vi "St temp.vi"(11 "Station Name":string) -> ()   [LabVIEW 2019]
uses:
  Ctrl/Conveyor Action.ctl
  <vilib>/Utility/miscctls.llb/LVPointTypeDef.ctl
  LLB/Message/Ctrl/MsgDataInput.ctl
  LLB/Message/Ctrl/MsgPageSelect.ctl
  LLB/Message/Ctrl/LogType.ctl
  Ctrl/Auto Inspection Station Name2.ctl
  Ctrl/Auto Inspection Data Name.ctl
  ab69a899-d2ec-4c26-af5e-ed1cd18d461c.vi
  9b7d8055-4de2-48cf-bbcb-f861e34e7884.vi
  2931b48d-cced-43b2-9067-584d882f955d.vi
  Function/Axis/Axis_Class/SubVI/Axis Motion/Axis_Go Home.vi
  <vilib>/JDP Science/JSONtext/JSON text to Variant.vi
  <vilib>/JDP Science/JSONtext/Variant to JSON Text.vi
  LLB/Commonly VI.lvlib
  LLB/Message/MsgShowAndLog.lvlib
panel:
  in  "Btn_Home":bool
  in  "AI":T1
  in  "Tab Control":enum32{"Page 1", "Page 2"}(tab)
  in  "CurrentAction":string
  in  "Status":string
  in  "Errset":bool
  out "Message":string
  out "Ring":u16(ring)
  in  "Btn_AutoRun":bool
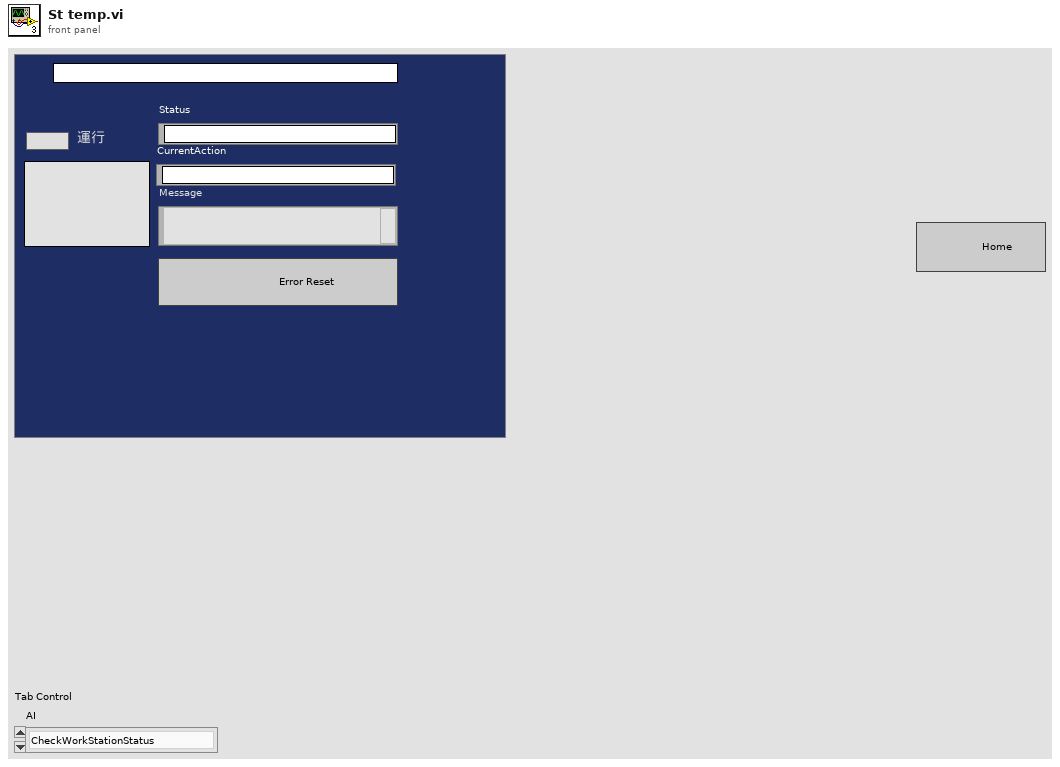
[diagram p1: front panel]
types:
  T1 = typedef "Conveyor Action.ctl" = enum16{"CheckWorkStationStatus", "Request Item In", "Check Product Ready In", "Wait Item In", "Check SlowSignal And Slow", "Check Arrive", "Rise Tray", "FixTray", "Imform Robot", "Wait Robot Imform", "DropTray Imform Out", "Wait Request ", "Flow Out"}
  T2 = enum8{"Enabled", "Disabled", "Disabled and Grayed Out"}
  T3 = typedef "LVPointTypeDef.ctl" = cluster{"Horizontal":i16, "Vertical":i16}
  T4 = typedef "MsgDataInput.ctl" = cluster{"MsgPageSelect":T5, "LogType":T6, "Msg":string, "Time":string}
  T5 = typedef "MsgShowAndLog.lvlib/MsgPageSelect.ctl" = enum16{"System", "Comm", "IO", "Action", "Alarm"}
  T6 = typedef "MsgShowAndLog.lvlib/LogType.ctl" = enum16{"Auto", "Manual", "Handshake", "Error"}
  T7 = typedef "Auto Inspection Station Name2.ctl" = enum16{"S1Barcode", "S2Measure", "S3Measure", "S4Measure", "S5Measure", "S11_LaserCheck", "S8_Vision AI"}
  T8 = typedef "Auto Inspection Data Name.ctl" = enum16{"LocalRun", "ItemSN(TimeCode)", "CurrentAction", "Error", "Data", "OKNG", "電壓值", "電壓值判斷", "電流值", "電流值判斷", "Laser1 Data", "Laser2 Data", "Laser OKNG", "StationNO"}
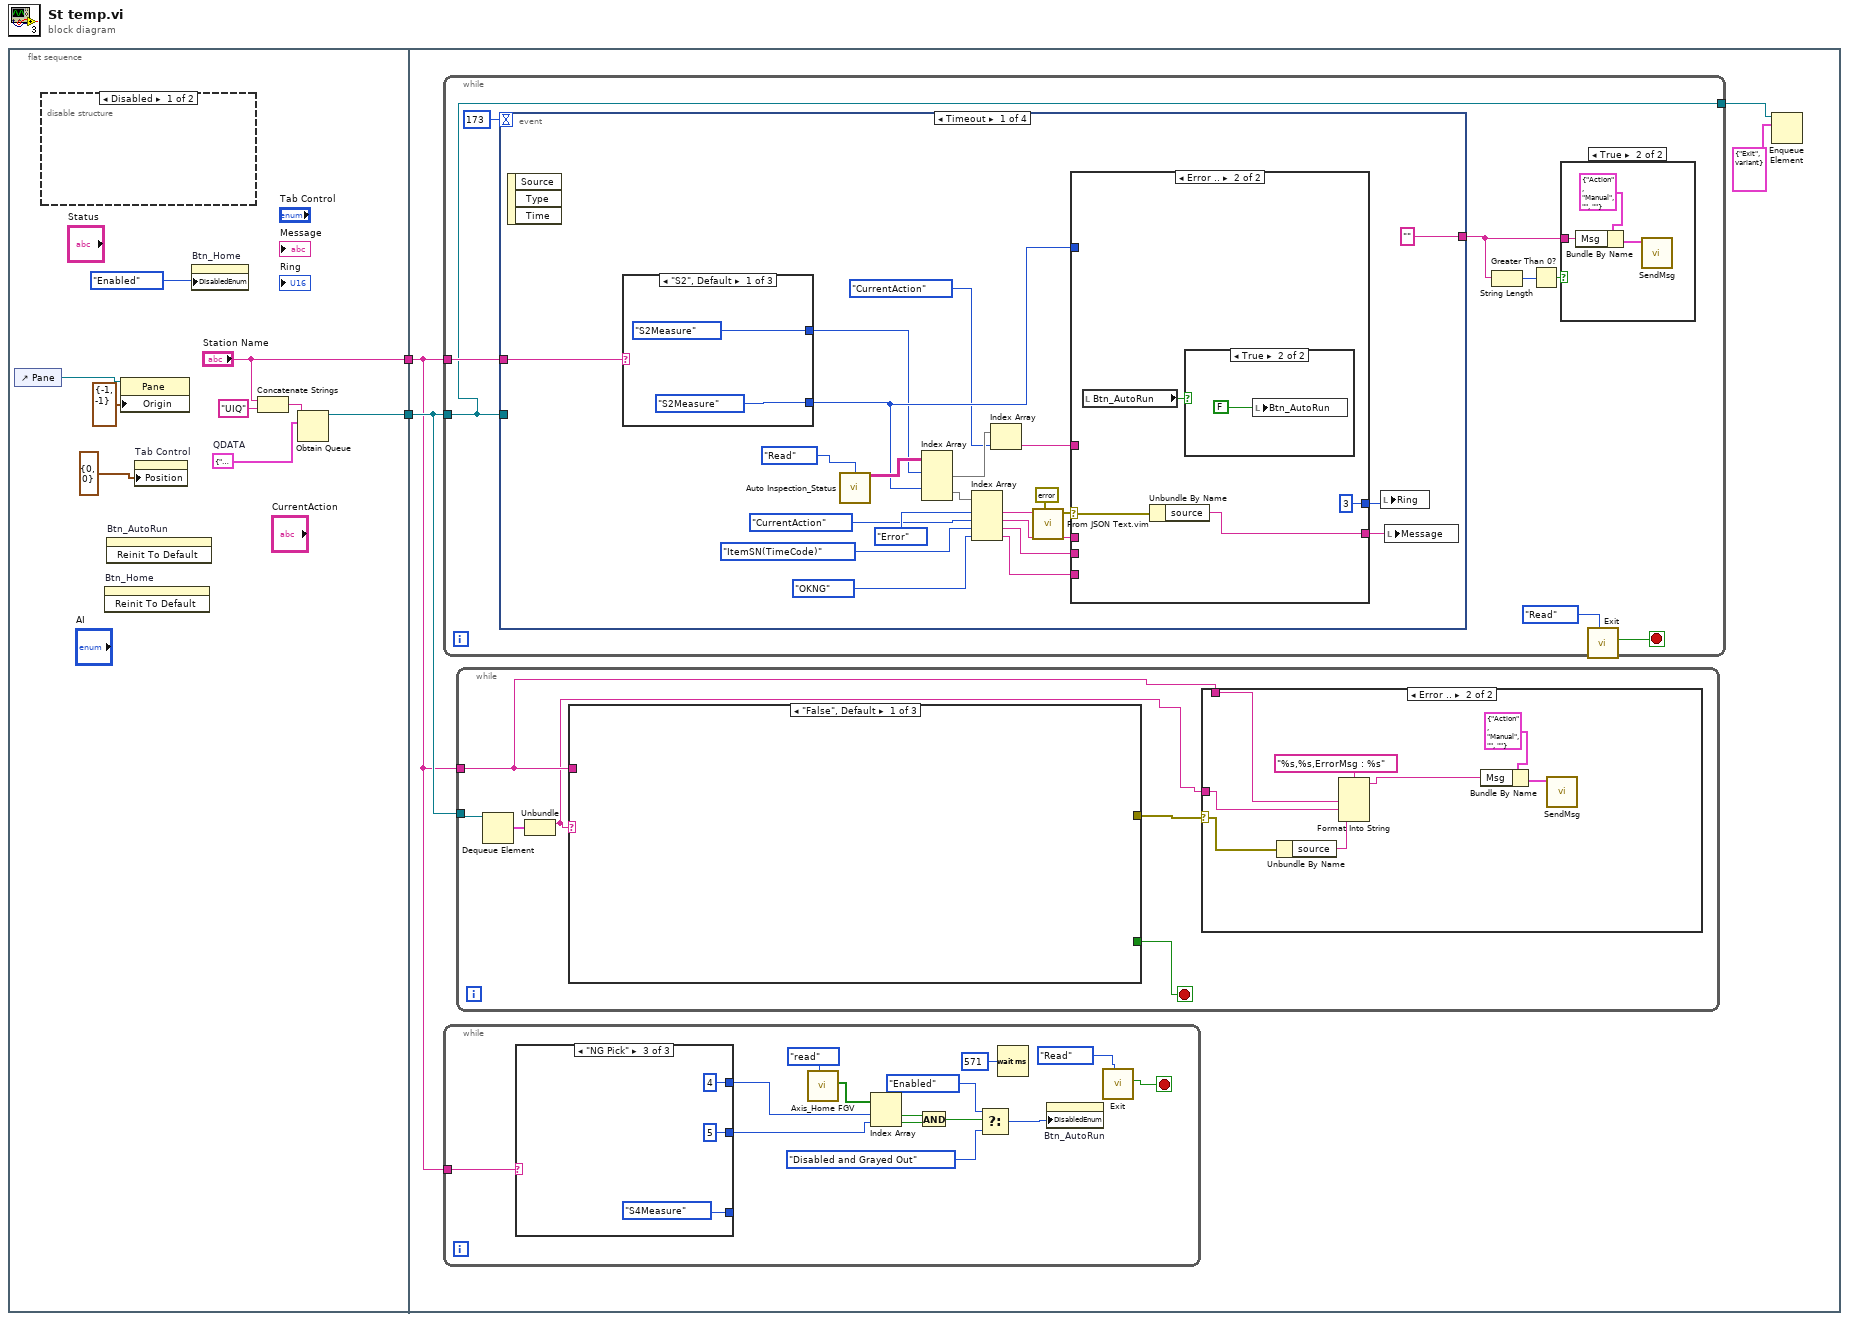
[diagram p0: block diagram]
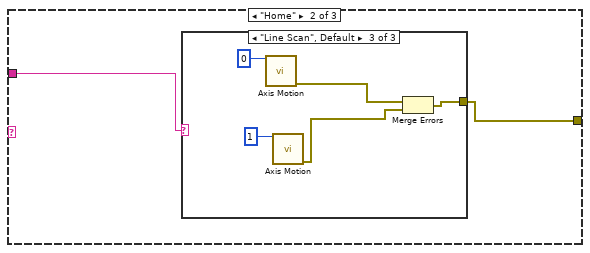
[diagram p4: hidden frame]
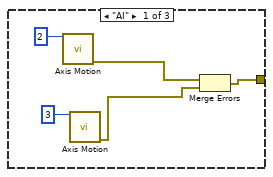
[diagram p5: hidden frame]
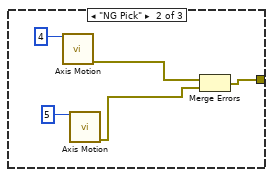
[diagram p6: hidden frame]
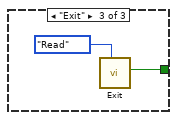
[diagram p7: hidden frame]
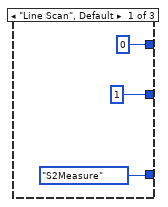
[diagram p8: hidden frame]
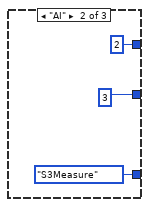
[diagram p9: hidden frame]
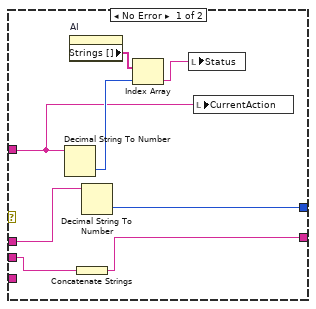
[diagram p11: hidden frame]
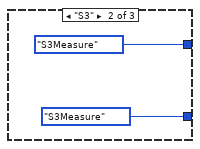
[diagram p13: hidden frame]
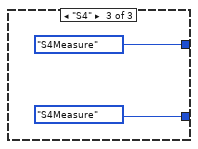
[diagram p14: hidden frame]
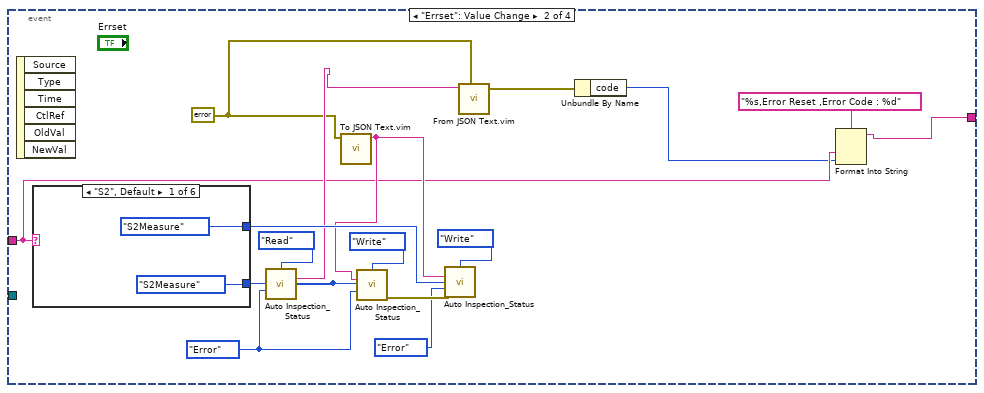
[diagram p15: hidden frame]
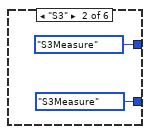
[diagram p16: hidden frame]
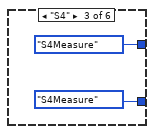
[diagram p17: hidden frame]
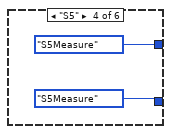
[diagram p18: hidden frame]
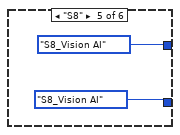
[diagram p19: hidden frame]
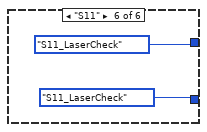
[diagram p20: hidden frame]
diagram:
  n1 = flat-sequence {
    tunnel: ["Station Name"] -> w2
    tunnel: [w3] -> w1
    tunnel: w2 -> [w12]
    tunnel: w1 -> [w15]
    frame #0 {
      w4 = cluster{"ACT":string, "DATA":variant} {"ACT"="", "DATA"=variant}  # QDATA
      n2 = control-ref of="Pane"() -> (w11:refnum<vi>)
      n3 = disable-structure shown="Disabled" {
        frame Disabled {
        }
        frame Enabled {
        }
      }
      n4 = invoke on="Btn_Home" class="Bool" method="Reinit To Default"() -> ()  [unwired: 3 in, 3 out]
      n5 = invoke on="Btn_AutoRun" class="Bool (strict)" method="Reinit To Default"() -> ()  [unwired: 3 in, 3 out]
      n6 = property class="Pane"(reference=w11, "Origin"=T3 {"Horizontal"=-1, "Vertical"=-1}) -> ()  [unwired: 1 in, 2 out]
      n7 = property on="Tab Control" class="TabCtl (strict)"("Position"=T3 {"Horizontal"=0, "Vertical"=0} ("Origin")) -> ()  [unwired: 2 in, 2 out]
      n8 = property on="Btn_Home" class="Bool"("DisabledEnum"=T2."Enabled" ("Disabled")) -> ()  [unwired: 2 in, 2 out]
      n9 = Concatenate Strings("Station Name", "UIQ" ("string")) -> (w5:string)
      n10 = Obtain Queue(name (unnamed)=w5, element data type=w4) -> (queue out=w3:refnum<queue>)  [unwired: 3 in, 2 out]
    }
    frame #1 {
      n11 = while {
        tunnel: w12 -> [w76]
        tunnel: w15 -> [w75]
        tunnel: [w75] -> w14
        stop <- w78 stop-if-true
        n12 = event shown="[0] Timeout" {
          selector: _ -> [_ _ _ _]
          dyn-events: _ -> [_ _ _ _]
          timeout: 173 -> [_ _ _ _]
          tunnel: w76 -> [w103 w126 w153 w186]
          tunnel: w75 -> [_ _ _ w185]
          tunnel: ["" w124 w155 w188] -> w74
          event Timeout {
            n13 = event-data() -> ()  [unwired: 1 in, 3 out]
            n14 = case shown="\"S2\", Default" w103 {
              tunnel: [Auto_Inspection_Station_Name2."S2Measure" ("Station") Auto_Inspection_Station_Name2."S3Measure" ("Station") Auto_Inspection_Station_Name2."S4Measure" ("Station")] -> w89
              tunnel: [Auto_Inspection_Station_Name2."S2Measure" ("Station") Auto_Inspection_Station_Name2."S3Measure" ("Station") Auto_Inspection_Station_Name2."S4Measure" ("Station")] -> w88
              frame "S2", Default {
              }
              frame "S3" {
              }
              frame "S4" {
              }
            }
            n15 = call "Auto Inspection_Status.vi"("Action"=enum16{"Initial", "Write", "Read"}."Read") -> ("Table Control"=w102:string[][])  [unwired: 12 in, 2 out]
            n16 = Index Array(array=w102, index (row) #1=w88, index (row) #2=w89) -> (element #1=w87:string[], element #2=w101:string[])  [unwired: 2 in]
            n17 = Index Array(array=w101, index #1=Auto_Inspection_Data_Name."Error" ("Data"), index #2=Auto_Inspection_Data_Name."CurrentAction" ("Data"), index #3=Auto_Inspection_Data_Name."ItemSN(TimeCode)" ("Data"), index #4=Auto_Inspection_Data_Name."OKNG" ("Data")) -> (element #1=w98:string, element #2=w95:string, element #3=w91:string, element #4=w83:string)
            n18 = Index Array(array=w87, index=Auto_Inspection_Data_Name."CurrentAction" ("Data")) -> (element=w85:string)
            n19 = call "From JSON Text.vim"("Data Type and Default Value"=errorcluster {"status"=FALSE, "code"=0, "source"=""} ("error constant"), "JSON"=w98) -> ("Data out"=w96:errorcluster)  [unwired: 8 in, 1 out]
            n20 = case shown="Error .." w96 {
              selector: w96 -> [_ w115]
              tunnel: w95 -> [w112 _]
              tunnel: [w111 3] -> w94
              tunnel: [w105 w114] -> w92
              tunnel: w91 -> [w106 _]
              tunnel: w89 -> [_ _]
              tunnel: w85 -> [w107 _]
              tunnel: w83 -> [_ _]
              frame No Error {
                n21 = Decimal String To Number(string=w107) -> (number=w109:i32)  [unwired: 2 in, 1 out]
                n22 = property on="AI" class="Enum (strict)"() -> ("Strings []"=w110:string[])  [unwired: 2 in, 2 out]
                n23 = Concatenate Strings(w106) -> (w105:string)
                n24 = Decimal String To Number(string=w112) -> (number=w111:i32)  [unwired: 2 in, 1 out]
                n25 = Index Array(array=w110, index=w109) -> (element=w108:string)
                n26 = local write "Status"(w108) -> ()
                n27 = local write "CurrentAction"(w107) -> ()
              }
              frame Error {
                n28 = local read "Btn_AutoRun"() -> (w113:bool)
                n29 = Unbundle By Name(w115) -> ("source"=w114:string)
                n30 = case shown="True" w113 {
                  frame False {
                  }
                  frame True {
                    n31 = local write "Btn_AutoRun"(FALSE) -> ()
                  }
                }
              }
            }
            n32 = local write "Ring"(w94) -> ()
            n33 = local write "Message"(w92) -> ()
          }
          event "Errset": Value Change {
            w128 = errorcluster {"status"=FALSE, "code"=0, "source"=""} ("error constant")
            w130 = Auto_Inspection_Data_Name."Error" ("Data")
            n34 = event-data() -> ()  [unwired: 1 in, 6 out]
            n35 = case shown="\"S2\", Default" w126 {
              tunnel: [Auto_Inspection_Station_Name2."S2Measure" ("Station") Auto_Inspection_Station_Name2."S3Measure" ("Station") Auto_Inspection_Station_Name2."S4Measure" ("Station") Auto_Inspection_Station_Name2."S5Measure" ("Station") Auto_Inspection_Station_Name2."S8_Vision AI" ("Station") Auto_Inspection_Station_Name2."S11_LaserCheck" ("Station")] -> w131
              tunnel: [Auto_Inspection_Station_Name2."S2Measure" ("Station") Auto_Inspection_Station_Name2."S3Measure" ("Station") Auto_Inspection_Station_Name2."S4Measure" ("Station") Auto_Inspection_Station_Name2."S5Measure" ("Station") Auto_Inspection_Station_Name2."S8_Vision AI" ("Station") Auto_Inspection_Station_Name2."S11_LaserCheck" ("Station")] -> w136
              frame "S2", Default {
              }
              frame "S3" {
              }
              frame "S4" {
              }
              frame "S5" {
              }
              frame "S8" {
              }
              frame "S11" {
              }
            }
            n36 = call "Auto Inspection_Status.vi"("Action"=enum16{"Initial", "Write", "Read"}."Read", "Station"=w131, "Data"=w130) -> ("DataOut"=w129:string)  [unwired: 10 in, 2 out]
            n37 = call "To JSON Text.vim"("Anything"=w128) -> ("<JSON>"=w134:string)  [unwired: 9 in, 1 out]
            n38 = call "Auto Inspection_Status.vi"("Action"=enum16{"Initial", "Write", "Read"}."Write", "DataIn"=w134, "Station"=w131, "Data"=w130) -> ("error out"=w137:errorcluster)  [unwired: 9 in, 2 out]
            n39 = call "Auto Inspection_Status.vi"("Action"=enum16{"Initial", "Write", "Read"}."Write", "DataIn"=w134, "Station"=w136, "Data"=Auto_Inspection_Data_Name."Error", "error in"=w137) -> ()  [unwired: 8 in, 3 out]
            n40 = call "From JSON Text.vim"("Data Type and Default Value"=w128, "JSON"=w129) -> ("Data out"=w127:errorcluster)  [unwired: 8 in, 1 out]
            n41 = Unbundle By Name(w127) -> ("code"=w125:i32)
            n42 = Format Into String(format string="%s,Error Reset ,Error Code : %d", w126, w125) -> (resulting string=w124:string)  [unwired: 2 in, 1 out]
          }
          event "Btn_AutoRun": Value Change {
            w159 = Auto_Inspection_Data_Name."LocalRun" ("Data")
            n43 = event-data() -> ("NewVal"=w152:bool)  [unwired: 1 in, 5 out]
            n44 = case shown="\"S2\", Default" w153 {
              tunnel: [Auto_Inspection_Station_Name2."S1Barcode" ("Station") Auto_Inspection_Station_Name2."S2Measure" ("Station") Auto_Inspection_Station_Name2."S3Measure" ("Station") Auto_Inspection_Station_Name2."S4Measure" ("Station") Auto_Inspection_Station_Name2."S8_Vision AI" ("Station") Auto_Inspection_Station_Name2."S11_LaserCheck" ("Station")] -> w160
              tunnel: [Auto_Inspection_Station_Name2."S1Barcode" ("Station") Auto_Inspection_Station_Name2."S2Measure" ("Station") Auto_Inspection_Station_Name2."S3Measure" ("Station") Auto_Inspection_Station_Name2."S4Measure" ("Station") Auto_Inspection_Station_Name2."S8_Vision AI" ("Station") Auto_Inspection_Station_Name2."S11_LaserCheck" ("Station")] -> w156
              frame "S1" {
              }
              frame "S2", Default {
              }
              frame "S3" {
              }
              frame "S4" {
              }
              frame "S8" {
              }
              frame "S11" {
              }
            }
            n45 = Select(t="1", s=w152, f="0") -> (s? t:f=w157:string)
            n46 = Select(t=T2."Disabled and Grayed Out" ("Disabled"), s=w152, f=T2."Enabled" ("Disabled")) -> (s? t:f=w164:T2)
            n47 = property on="Btn_Home" class="Bool"("DisabledEnum"=w164) -> ()  [unwired: 2 in, 2 out]
            n48 = call "Auto Inspection_Status.vi"("Action"=enum16{"Initial", "Write", "Read"}."Write", "DataIn"=w157, "Station"=w160, "Data"=w159) -> ("error out"=w158:errorcluster)  [unwired: 9 in, 2 out]
            n49 = disable-structure shown="Enabled" {
              disable-tunnel: w159 -> [w170 _]
              disable-tunnel: w158 -> [w169 _]
              disable-tunnel: w157 -> [w168 _]
              disable-tunnel: w156 -> [w167 _]
              frame Disabled {
                n50 = call "Auto Inspection_Status.vi"("Action"=enum16{"Initial", "Write", "Read"}."Write", "DataIn"=w168, "Station"=w167, "Data"=w170, "error in"=w169) -> ()  [unwired: 8 in, 3 out]
              }
              frame Enabled {
              }
            }
            n51 = Format Into String(format string="%s,Auto Run,%s", w153, w152) -> (resulting string=w155:string)  [unwired: 2 in, 1 out]
          }
          event "Btn_Home": Value Change {
            n52 = event-data() -> ()  [unwired: 1 in, 6 out]
            n53 = Enqueue Element(queue=w185, element=cluster{"ACT":string, "DATA":variant} {"ACT"="Home", "DATA"=variant}) -> ()  [unwired: 2 in, 3 out]
            n54 = Format Into String(format string="%s,Search HM", w186) -> (resulting string=w188:string)  [unwired: 2 in, 1 out]
          }
        }
        n55 = String Length(string=w74) -> (length=w73:i32)
        n56 = Greater Than 0?(x=w73) -> (x > 0?=w72:bool)
        n57 = case shown="True" w72 {
          tunnel: w74 -> [_ w80]
          frame False {
          }
          frame True {
            n58 = Bundle By Name(cluster=T4 {"MsgPageSelect"=enum."Action", "LogType"=enum."Manual", "Msg"="", "Time"=""} ("DataIn"), "Msg"=w80) -> (w81:T4)
            n59 = call "SendMsg.vi"("DataIn"=w81) -> ()  [unwired: 10 in, 1 out]
          }
        }
        n60 = call "Exit.vi"("Enum"=enum16{"Initial", "Read", "Write"}."Read") -> ("ExitOut"=w78:bool)  [unwired: 10 in]
      }
      n61 = while {
        tunnel: w12 -> [w60]
        stop <- w62 stop-if-true
        n62 = case shown="\"NG Pick\"" w60 {
          tunnel: [Auto_Inspection_Station_Name2."S2Measure" ("Station") Auto_Inspection_Station_Name2."S3Measure" ("Station") Auto_Inspection_Station_Name2."S4Measure" ("Station")] -> _
          tunnel: [0 2 4] -> w57
          tunnel: [1 ("Axis") 3 5 ("Axis")] -> w56
          frame "Line Scan", Default {
          }
          frame "AI" {
          }
          frame "NG Pick" {
          }
        }
        n63 = call "Axis_Home FGV.vi"("Enum"=enum16{"Initial", "write", "read"}."read") -> ("HMSStatus"=w58:bool[])  [unwired: 9 in, 1 out]
        n64 = Index Array(array=w58, index #1=w57, index #2=w56) -> (element #1=w54:bool, element #2=w55:bool)
        n65 = And(x=w54, y=w55) -> (x .and. y?=w53:bool)
        n66 = Select(t=T2."Enabled" ("Disabled"), s=w53, f=T2."Disabled and Grayed Out" ("Disabled")) -> (s? t:f=w49:T2)
        n67 = Wait (ms)(milliseconds to wait=u32 571) -> ()  [unwired: 1 out]
        n68 = property on="Btn_AutoRun" class="Bool (strict)"("DisabledEnum"=w49) -> ()  [unwired: 2 in, 2 out]
        n69 = call "Exit.vi"("Enum"=enum16{"Initial", "Read", "Write"}."Read") -> ("ExitOut"=w62:bool)  [unwired: 10 in]
      }
      n70 = while {
        tunnel: w15 -> [w21]
        tunnel: w12 -> [w17]
        stop <- w19 stop-if-true
        n71 = Dequeue Element(queue=w21) -> (element=w20:cluster{"ACT":string, "DATA":variant})  [unwired: 2 in, 3 out]
        n72 = Unbundle(w20) -> ("ACT"=w16:string)  [unwired: 1 out]
        n73 = case shown="\"False\", Default" w16 {
          tunnel: [_ _ w47] -> w19
          tunnel: w17 -> [_ w31 _]
          tunnel: [_ w30 _] -> w18
          frame "False", Default {
          }
          frame "Home" {
            n74 = case shown="\"Line Scan\", Default" w31 {
              tunnel: [w32 w37 w42] -> w30
              frame "AI" {
                n75 = call-poly "Axis Motion.vi"("Axis Index"=2) -> ("error"=w34:errorcluster)  [unwired: 10 in]
                n76 = call-poly "Axis Motion.vi"("Axis Index"=3) -> ("error"=w33:errorcluster)  [unwired: 10 in]
                n77 = Merge Errors(w34, w33) -> (w32:errorcluster)
              }
              frame "NG Pick" {
                n78 = call-poly "Axis Motion.vi"("Axis Index"=4) -> ("error"=w39:errorcluster)  [unwired: 10 in]
                n79 = call-poly "Axis Motion.vi"("Axis Index"=5) -> ("error"=w38:errorcluster)  [unwired: 10 in]
                n80 = Merge Errors(w39, w38) -> (w37:errorcluster)
              }
              frame "Line Scan", Default {
                n81 = call-poly "Axis Motion.vi"("Axis Index"=0) -> ("error"=w44:errorcluster)  [unwired: 10 in]
                n82 = call-poly "Axis Motion.vi"("Axis Index"=1) -> ("error"=w43:errorcluster)  [unwired: 10 in]
                n83 = Merge Errors(w44, w43) -> (w42:errorcluster)
              }
            }
          }
          frame "Exit" {
            n84 = call "Exit.vi"("Enum"=enum16{"Initial", "Read", "Write"}."Read") -> ("ExitOut"=w47:bool)  [unwired: 10 in]
          }
        }
        n85 = case shown="Error .." w18 {
          selector: w18 -> [_ w23]
          tunnel: w17 -> [_ w25]
          tunnel: w16 -> [_ w24]
          frame No Error {
          }
          frame Error {
            n86 = Unbundle By Name(w23) -> ("source"=w22:string)
            n87 = Format Into String(format string="%s,%s,ErrorMsg : %s", w25, w24, w22) -> (resulting string=w26:string)  [unwired: 2 in, 1 out]
            n88 = Bundle By Name(cluster=T4 {"MsgPageSelect"=enum."Action", "LogType"=enum."Manual", "Msg"="", "Time"=""} ("DataIn"), "Msg"=w26) -> (w29:T4)
            n89 = call "SendMsg.vi"("DataIn"=w29) -> ()  [unwired: 10 in, 1 out]
          }
        }
      }
      n90 = Enqueue Element(queue=w14, element=cluster{"ACT":string, "DATA":variant} {"ACT"="Exit", "DATA"=variant}) -> ()  [unwired: 2 in, 3 out]
    }
  }
